vi "Write Wash Step Selection Buttons.vi"(10 "Wash Step Selection Buttons":refnum<vi>, 11 "Entry Console Start Msg in":refnum<class "Register Entry Console References.lvclass">) -> (3 "Entry Console Start Msg out":refnum<class "Register Entry Console References.lvclass">)   [LabVIEW 2012, in "Car Wash Controller.lvlib" / "Register Entry Console References.lvclass"]
uses:
  Register Entry Console References.lvclass
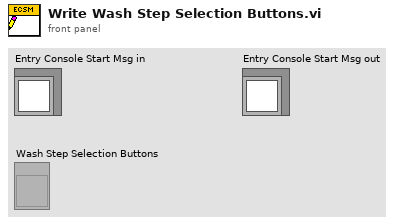
[diagram p1: front panel]
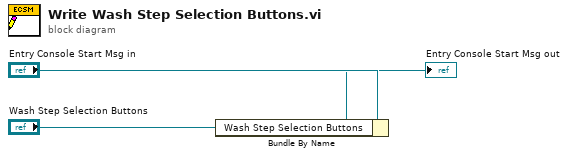
[diagram p0: block diagram]
diagram:
  n1 = Bundle By Name(cluster="Entry Console Start Msg in", "Wash Step Selection Buttons"="Wash Step Selection Buttons") -> (→"Entry Console Start Msg out":refnum<class "Register Entry Console References.lvclass">)
